vi "Write Step Config.vi"(8 "error in (no error)":errorcluster, 10 "Test Config":T1, 11 "Test 1 in":refnum<class "Measure.lvclass">) -> (0 "error out":errorcluster, 3 "Test 1 out":refnum<class "Measure.lvclass">)   [LabVIEW 2021, in "Sequence Engine.lvlib" / "Measure.lvclass"]
uses:
  Measure.lvclass
  Step Factory/Test Config.ctl
  Measure.lvclass/Measure.ctl
  Step Factory/Test Factory.lvclass
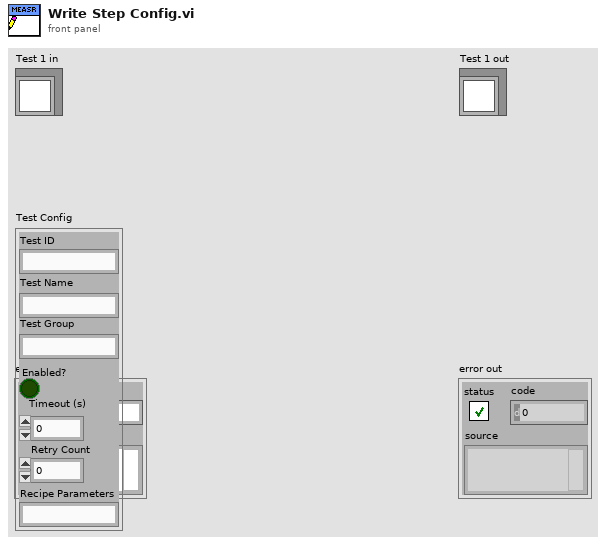
[diagram p1: front panel]
types:
  T1 = typedef "Sequence Engine.lvlib/Test Factory.lvclass/Test Config.ctl" = cluster{"Test ID":string, "Test Name":string, "Test Group":string, "Enabled?":bool, "Timeout (s)":u16, "Retry Count":u16, "Recipe Parameters":string}
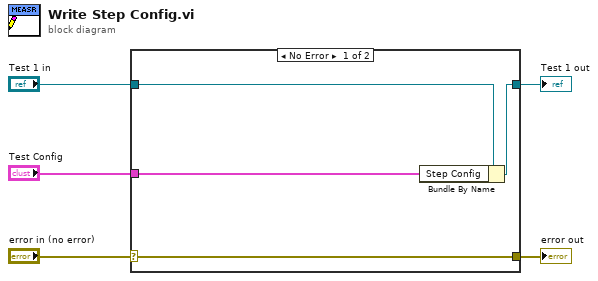
[diagram p0: block diagram]
diagram:
  n1 = case shown="No Error" "error in (no error)" {
    selector: "error in (no error)" -> [w9 w10]
    tunnel: [w9 w10] -> w4
    tunnel: [w7 w11] -> w2
    tunnel: "Test 1 in" -> [w8 w11]
    tunnel: "Test Config" -> [w6 _]
    frame No Error {
      n2 = Bundle By Name(cluster=w8, "Step Config"=w6) -> (w7:refnum<class "Measure.lvclass">)
    }
    frame Error {
    }
  }
  "error out" <- w4
  "Test 1 out" <- w2
